vi "error event gen.vi"(0 "error in (no error)":errorcluster) -> (1 "Error event":refnum<user-event>, 2 "error out":errorcluster)   [LabVIEW 2010, in "ErrorLog.lvlib"]
doc: "This VI serves to fire an event that logs the error to a log file via the shell.\nCustom error codes and their descriptions can be input via the error global variables or read from an error file.\nThe first execution creates the user event and subsequent errors are logged.\n\nInputs:\nError in - error input cluster (to be logged)\n\nOutputs:\nError out - error output cluster (duplicate of input cluster for further program usage)"
uses:
  ErrorLog.lvlib
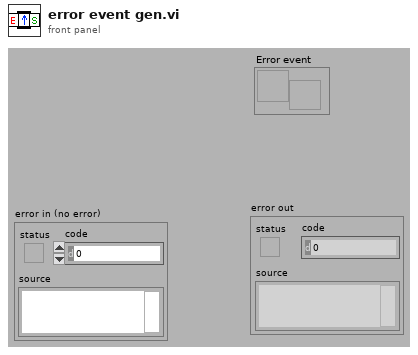
[diagram p1: front panel]
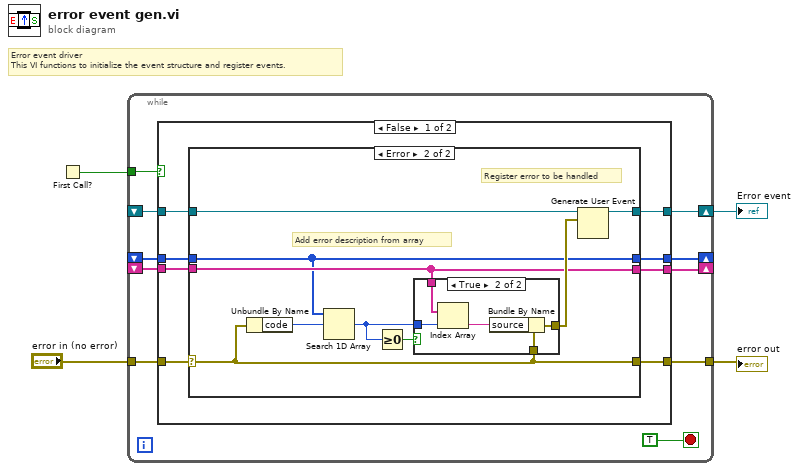
[diagram p0: block diagram]
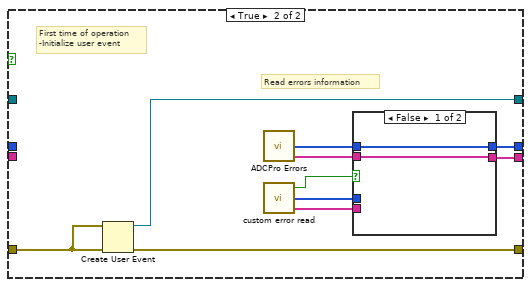
[diagram p4: hidden frame]
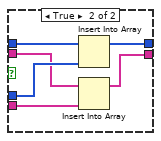
[diagram p5: hidden frame]
diagram:
  # "Error event driver\nThis VI functions to initialize the event structure and register events."
  n1 = First Call?() -> (First Call?: T/F=w4:bool)
  n2 = while {
    shift-right: [w12] -> w3
    shift-left: _ -> [w14]
    tunnel: w4 -> [w13]
    tunnel: "error in (no error)" -> [w10]
    tunnel: [w9] -> w1
    shift-right: [w7] -> _
    shift-left: _ -> [w8]
    shift-right: [w6] -> _
    shift-left: _ -> [w5]
    stop <- TRUE stop-if-true
    n3 = case shown="False" w13 {
      tunnel: w14 -> [w22 _]
      tunnel: w10 -> [w19 w49]
      tunnel: [w21 w51] -> w9
      tunnel: [w20 w50] -> w12
      tunnel: w8 -> [w18 _]
      tunnel: [w17 w47] -> w7
      tunnel: [w15 w42] -> w6
      tunnel: w5 -> [w16 _]
      frame False {
        n4 = case shown="Error" w19 {
          selector: w19 -> [w25 w31]
          tunnel: w22 -> [w26 w35]
          tunnel: [w25 w31] -> w21
          tunnel: [w26 w34] -> w20
          tunnel: w18 -> [w24 w29]
          tunnel: [w24 w29] -> w17
          tunnel: w16 -> [w23 w30]
          tunnel: [w23 w30] -> w15
          frame No Error {
            # "No error"
          }
          frame Error {
            # "Add error description from array"
            # "Register error to be handled"
            n5 = Unbundle By Name(w31) -> ("code"=w33:i32)
            n6 = Search 1D Array(1D array=w29, element=w33) -> (index of element=w28:i32)  [unwired: 1 in]
            n7 = Greater Or Equal To 0?(x=w28) -> (x >= 0?=w27:bool)
            n8 = case shown="True" w27 {
              tunnel: [w36 w40] -> w32
              tunnel: w31 -> [w36 w39]
              tunnel: w30 -> [_ w38]
              tunnel: w28 -> [_ w37]
              frame False {
              }
              frame True {
                n9 = Index Array(array=w38, index=w37) -> (element=w41:string)
                n10 = Bundle By Name(cluster=w39, "source"=w41) -> (w40:errorcluster)
              }
            }
            n11 = Generate User Event(user event=w35, event data cluster=w32) -> (user event out=w34:refnum<user-event>)  [unwired: 1 in, 1 out]
          }
        }
      }
      frame True {
        # "Read errors information"
        # "First time of operation\n-Initialize user event"
        n12 = Create User Event(user event datatype=w49, error in=w49) -> (user event=w50:refnum<user-event>, error out=w51:errorcluster)
        n13 = call "ADCPro Errors.vi"() -> ("Error Description - Custom"=w48:string[], "Error Codes - Custom"=w45:i32[])  [unwired: 4 in]
        n14 = call "custom error read.vi"() -> ("Description"=w43:string[], "Codes"=w44:i32[], "file or folder exists?"=w46:bool)  [unwired: 3 in]
        n15 = case shown="False" w46 {
          tunnel: w48 -> [w52 w54]
          tunnel: [w53 w56] -> w47
          tunnel: w45 -> [w53 w59]
          tunnel: w44 -> [_ w58]
          tunnel: w43 -> [_ w57]
          tunnel: [w52 w55] -> w42
          frame False {
          }
          frame True {
            n16 = Insert Into Array(array=w59, new element=w58) -> (w56:i32[])  [unwired: 1 in]
            n17 = Insert Into Array(array=w54, new element=w57) -> (w55:string[])  [unwired: 1 in]
          }
        }
      }
    }
  }
  "error out" <- w1
  "Error event" <- w3
